vi "createInstanceFromBuilder.vi"(8 "error in (no error)":errorcluster, 10 "IInstanceBuilder in":refnum<class "IInstanceBuilder.lvclass">, 11 "IInstance in":refnum<class "IInstance.lvclass">) -> (0 "error out":errorcluster, 3 "IInstance out":refnum<class "IInstance.lvclass">)   [LabVIEW 2022 SP3, in "openDAQ.lvlib" / "IBaseObject.lvlib" / "IPropertyObject.lvlib" / "IComponent.lvlib" / "IFolder.lvlib" / "IDevice.lvlib" / "IInstance.lvlib" / "IInstance.lvclass"]
uses:
  <instrlib>/openDAQ/Public/Classes/IInstance/IInstance.lvclass
  C:/Program Files (x86)/National Instruments/LabVIEW 2022/instr.lib/openDAQ/Public/Classes/IBaseObject/IBaseObject.lvclass
  <instrlib>/openDAQ/Public/Classes/IInstanceBuilder/IInstanceBuilder.lvclass
  <instrlib>/openDAQ/Public/Classes/IBaseObject/IBaseObject.lvclass/IBaseObject.ctl
  <instrlib>/openDAQ/Public/Classes/IBaseObject/Accessor/Read reference.vi
  <instrlib>/openDAQ/Public/Classes/IBaseObject/Accessor/Write reference.vi
  <instrlib>/openDAQ/Binaries/Windows/x86/copendaq32.dll
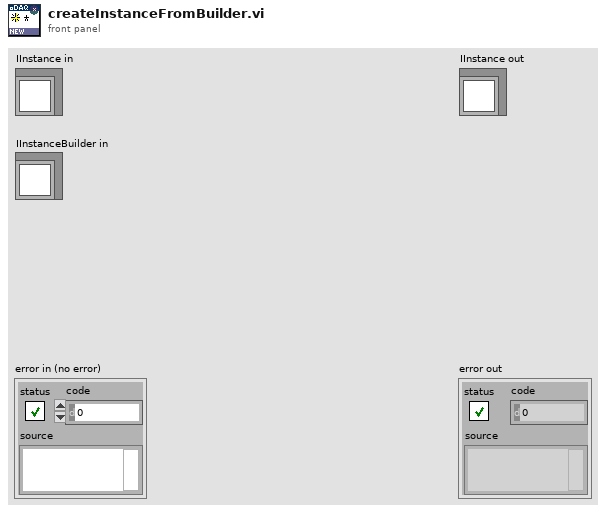
[diagram p1: front panel]
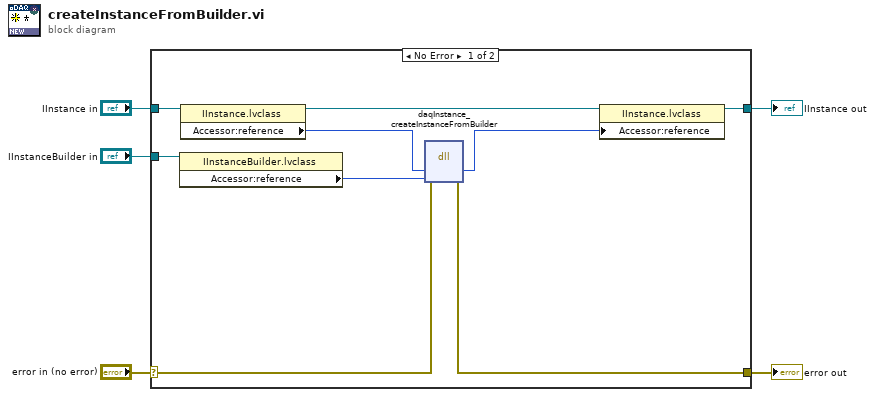
[diagram p0: block diagram]
diagram:
  n1 = case shown="No Error" "error in (no error)" {
    selector: "error in (no error)" -> [w11 w16]
    tunnel: [w6 w16] -> w4
    tunnel: [w12 w15] -> w2
    tunnel: "IInstance in" -> [w14 w15]
    tunnel: "IInstanceBuilder in" -> [w8 _]
    frame No Error {
      n2 = property class="IInstanceBuilder.lvclass"(reference=w8) -> ("Accessor:reference"=w7:i64)  [unwired: 1 in, 2 out]
      n3 = property class="IInstance.lvclass"(reference=w14) -> (reference out=w13:refnum<class "IInstance.lvclass">, "Accessor:reference"=w10:i64)  [unwired: 1 in, 1 out]
      n4 = dll-call lib="C:/Program Files (x86)/National Instruments/LabVIEW 2022/instr.lib/openDAQ/Binaries/Windows/x86/copendaq*.*" fn="daqInstance_createInstanceFromBuilder"(error in=w11, "instance"=w10, "builder"=w7) -> (error out=w6:errorcluster, "instance"=w9:i64)  [unwired: 4 in, 1 out]
      n5 = property class="IInstance.lvclass"(reference=w13, "Accessor:reference"=w9) -> (reference out=w12:refnum<class "IInstance.lvclass">)  [unwired: 1 in, 1 out]
    }
    frame Error {
    }
  }
  "error out" <- w4
  "IInstance out" <- w2
